vi "Test.vi"(0 "Limit_ni(mm)":dbl, 1 "XYGraphGN":refnum<vi>, 5 "拐点位移":dbl, 7 "曲线索引":i32, 9 "Limit_fi(mm)":dbl=21.5, 11 "limit":T1) -> (3 "ok？":bool, 4 "min(mm)":dbl, 6 "最大位移":bool, 8 "拐点压力":dbl, 10 "max(mm)":dbl, 12 "max(n)":dbl, 14 "数组":string[][](array[string]), 15 "最小位移":bool)   [LabVIEW 2017]
panel:
  out "XY_out":cluster{"S":dbl[], "F":dbl[]}[](graph)
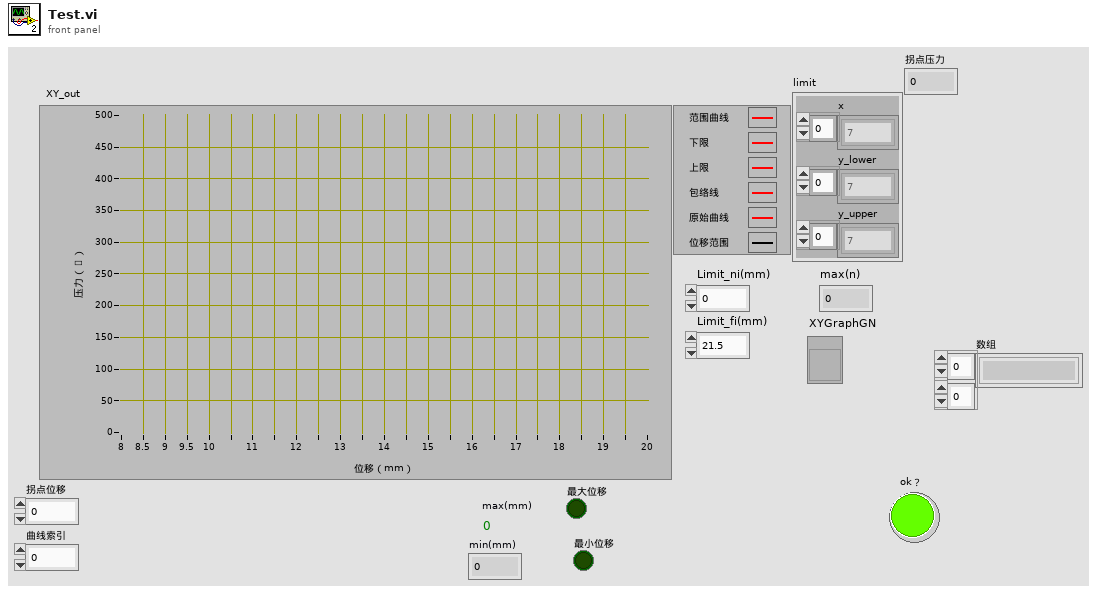
[diagram p1: front panel]
types:
  T1 = cluster{"x":dbl[], "y_lower":dbl[], "y_upper":dbl[]}
  T2 = cluster{cluster{dbl[], dbl[]}, cluster{"y1_upper":dbl, "y1_upper":dbl, "y1_upper":dbl, "y2_upper":dbl, "y2_upper":dbl, "y2_upper":dbl}}[]
  T3 = cluster{"y1_upper":dbl, "y1_upper":dbl, "y1_upper":dbl, "y2_upper":dbl, "y2_upper":dbl, "y2_upper":dbl}
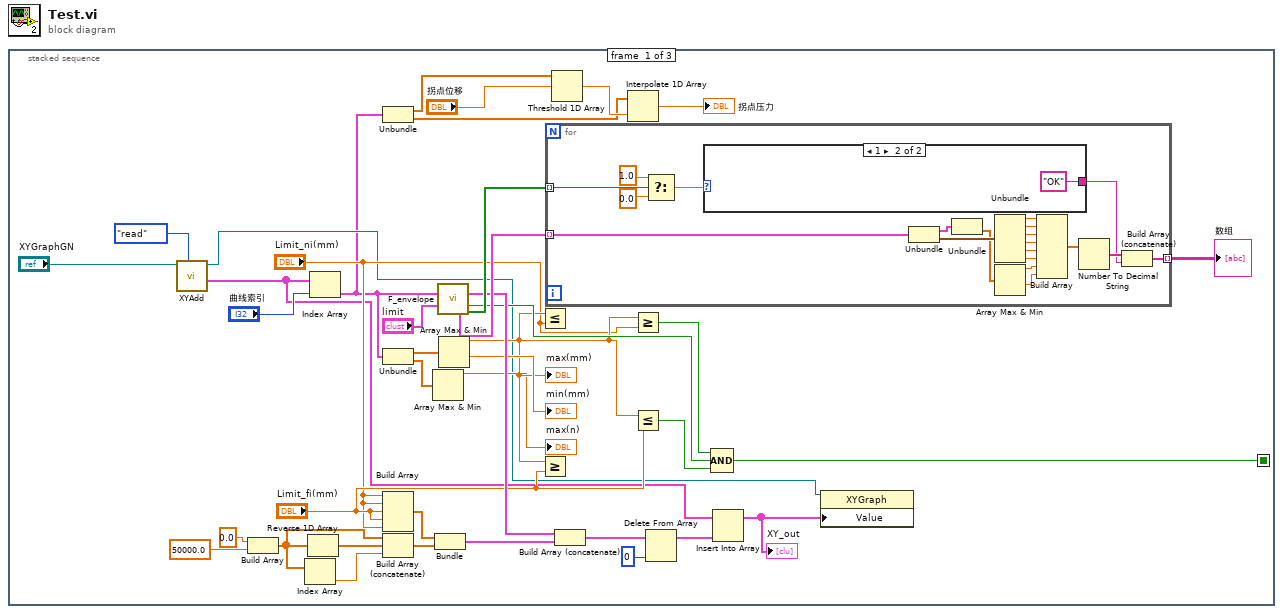
[diagram p0: block diagram]
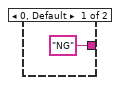
[diagram p2: hidden frame]
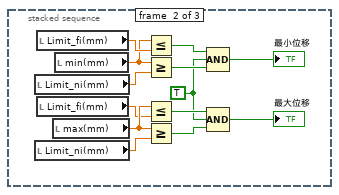
[diagram p3: hidden frame]
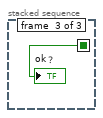
[diagram p4: hidden frame]
diagram:
  n1 = stacked-sequence {
    seq-local: [w2 _ _] -> [_ _ w75]
    frame #0 {
      n2 = call "XYAdd.vi"("枚举"=enum16{"insert", "add", "read", "reset"}."read", "XYGraph"="XYGraphGN") -> ("XYData"=w9:cluster{dbl[], dbl[]}[], "XYGraph 2"=w18:refnum<vi>)  [unwired: 8 in]
      n3 = Build Array(0.0 ("元素"), 50000.0 ("元素")) -> (w30:dbl[])
      n4 = Index Array(array=w30) -> (element=w32:dbl)  [unwired: 1 in]
      n5 = Reverse 1D Array(array=w30) -> (reversed array=w34:dbl[])
      n6 = Index Array(array=w9, index="曲线索引") -> (element=w17:cluster{dbl[], dbl[]})
      n7 = Unbundle(w17) -> (w16:dbl[], w13:dbl[])
      n8 = Unbundle(w17) -> (w36:dbl[], w20:dbl[])
      n9 = Build Array("Limit_ni(mm)", "Limit_ni(mm)", "Limit_fi(mm)", "Limit_fi(mm)", "Limit_ni(mm)") -> (w35:dbl[])
      n10 = Build Array (concatenate)(w30, w34, w32) -> (w33:dbl[])
      n11 = Array Max & Min(array=w20) -> (max value=→"max(n)":dbl)  [unwired: 3 out]
      n12 = Bundle(w35, w33) -> (w10:cluster{dbl[], dbl[]})  [unwired: 1 in]
      n13 = call "F_envelope.vi"("XY_in"=w17, "limit"="limit") -> ("XY_out"=w37:cluster{dbl[], dbl[]}[], "ok"=w25:bool, "interval_data_parameter"=w39:T2, "ok_all interval"=w38:bool[])  [unwired: 10 in]
      n14 = Array Max & Min(array=w36) -> (max value=w23:dbl, min value=→"min(mm)":dbl)  [unwired: 2 out]
      "max(mm)" <- w23
      n15 = Less Or Equal?(x=w23, y="Limit_ni(mm)") -> ()  [unwired: 1 out]
      n16 = Greater Or Equal?(x=w23, y="Limit_fi(mm)") -> ()  [unwired: 1 out]
      n17 = for {
        tunnel: w39 -> [w59] mode=indexing
        tunnel: w38 -> [w47] mode=indexing
        tunnel: [w41] -> w28 mode=indexing
        n18 = Select(t=1.0, s=w47, f=0.0 ("t")) -> (s? t:f=w44:dbl)
        n19 = case shown="1" w44 {
          tunnel: ["NG" "OK"] -> w40
          frame 0, Default {
          }
          frame 1 {
          }
        }
        n20 = Unbundle(w59) -> (w58:cluster{dbl[], dbl[]}, w57:T3)
        n21 = Unbundle(w58) -> (w56:dbl[])  [unwired: 1 out]
        n22 = Unbundle(w57) -> ("y1_upper"=w55:dbl, "y1_upper"=w54:dbl, "y1_upper"=w53:dbl, "y2_upper"=w52:dbl, "y2_upper"=w51:dbl, "y2_upper"=w50:dbl)
        n23 = Array Max & Min(array=w56) -> (max value=w49:dbl, min value=w48:dbl)  [unwired: 2 out]
        n24 = Build Array(w55, w54, w53, w52, w51, w50, w49, w48) -> (w43:dbl[])
        n25 = Number To Decimal String(number=w43) -> (decimal integer string=w42:string[])  [unwired: 1 in]
        n26 = Build Array (concatenate)(w42, w40) -> (w41:string[])
      }
      "数组" <- w28
      n27 = Threshold 1D Array(2:"拐点位移", 3:w16) -> (0:w14:dbl)  [unwired: 1 in]
      n28 = Build Array (concatenate)(w37, w10) -> (w8:cluster{dbl[], dbl[]}[])
      n29 = Interpolate 1D Array(1:w14, 2:w13) -> (0:→"拐点压力":dbl)
      n30 = Greater Or Equal?(x=w23, y="Limit_ni(mm)") -> (x >= y?=w4:bool)
      n31 = Less Or Equal?(x=w23, y="Limit_fi(mm)") -> (x <= y?=w3:bool)
      n32 = Delete From Array(array=w8, index=0 ("索引")) -> (array with subset deleted=w7:cluster{dbl[], dbl[]}[])  [unwired: 1 in, 1 out]
      n33 = Compound Arithmetic op=AND(w4, w25, w3) -> (w2:bool)
      n34 = Insert Into Array(array=w9, new element=w7) -> (w6:cluster{dbl[], dbl[]}[])  [unwired: 1 in]
      "XY_out" <- w6
      n35 = property class="XYGraph"(reference=w18, "Value"=w6) -> ()  [unwired: 1 in, 2 out]
    }
    frame #1 {
      w62 = TRUE ("值")
      n36 = local read "Limit_ni(mm)"() -> (w65:dbl)
      n37 = local read "Limit_ni(mm)"() -> (w71:dbl)
      n38 = local read "Limit_fi(mm)"() -> (w67:dbl)
      n39 = local read "Limit_fi(mm)"() -> (w70:dbl)
      n40 = local read "max(mm)"() -> (w74:dbl)
      n41 = local read "min(mm)"() -> (w66:dbl)
      n42 = Less Or Equal?(x=w66, y=w67) -> (x <= y?=w64:bool)
      n43 = Greater Or Equal?(x=w66, y=w65) -> (x >= y?=w73:bool)
      n44 = Less Or Equal?(x=w74, y=w70) -> (x <= y?=w72:bool)
      n45 = Greater Or Equal?(x=w74, y=w71) -> (x >= y?=w68:bool)
      n46 = Compound Arithmetic op=AND(w64, w62, w73) -> (→"最小位移":bool)
      n47 = Compound Arithmetic op=AND(w72, w62, w68) -> (→"最大位移":bool)
    }
    frame #2 {
      "ok？" <- w75
    }
  }
